vi "set_smith_axis_label.vi"(4 "r/x_scale":bool, 5 "left_center":dbl=300.0, 6 "show_z":bool=TRUE, 7 "top_center":dbl=300.0, 8 "Z50":dbl=50.0, 9 "x":dbl[](array[numeric])=[0.2, 0.4, 0.6, 0.8, 1.0, 1.2, 1.6, 2.0, 3.0, 5.0, -0.2, -0.4, -0.6, -0.8, -1.0, -1.2, -1.6, -2.0, -3.0, -5.0], 10 "r":dbl[](array[numeric])=[0.0, 0.1, 0.2, 0.3, 0.5, 0.7, 1.0, 1.4, 2.0, 3.0, 5.0, 10.0, 20.0], 11 "smith_in":picture) -> (3 "smith_out":picture)   [LabVIEW 2025]
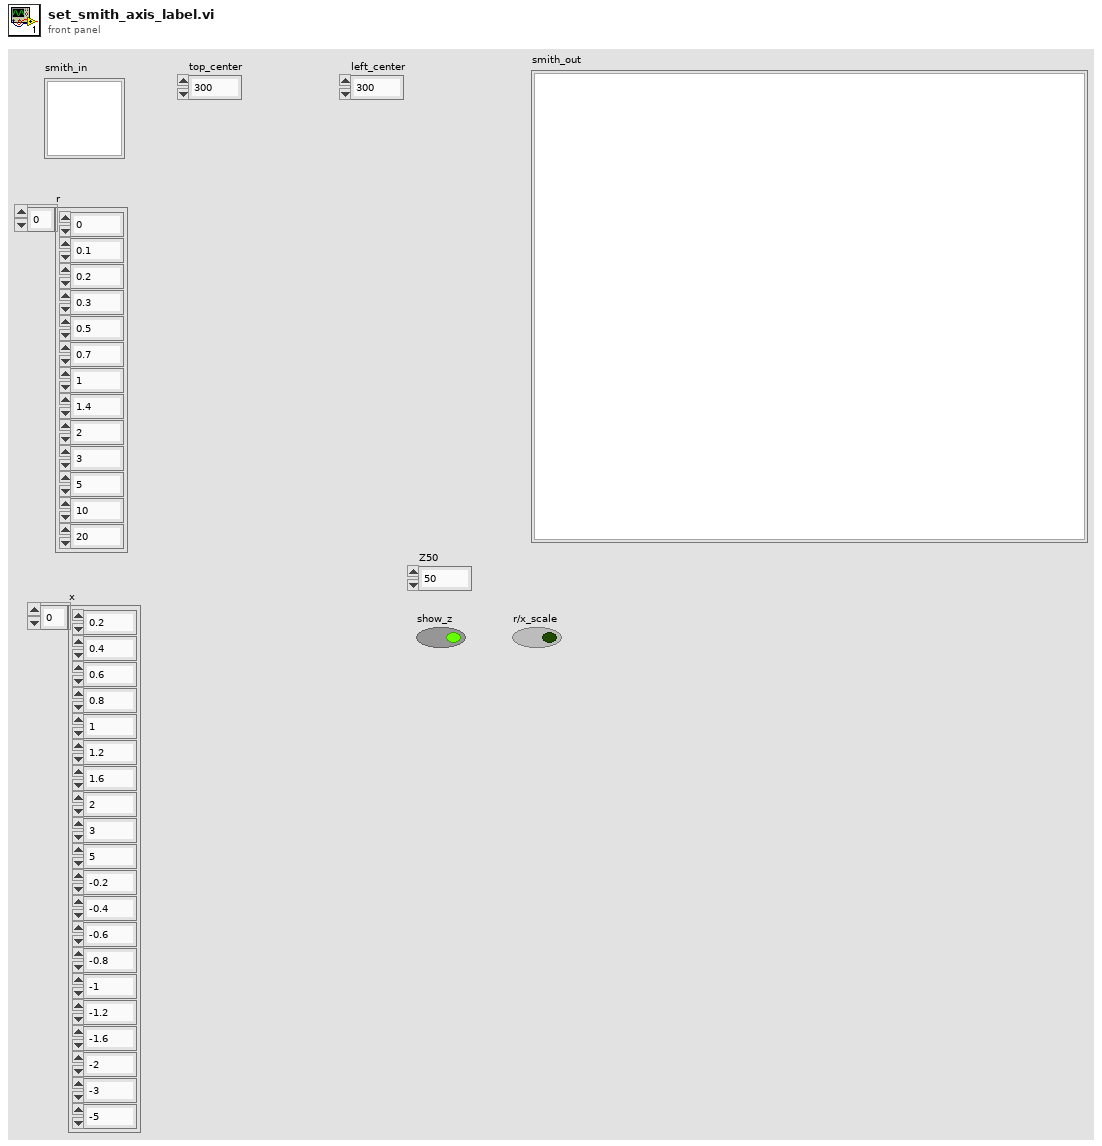
[diagram p1: front panel]
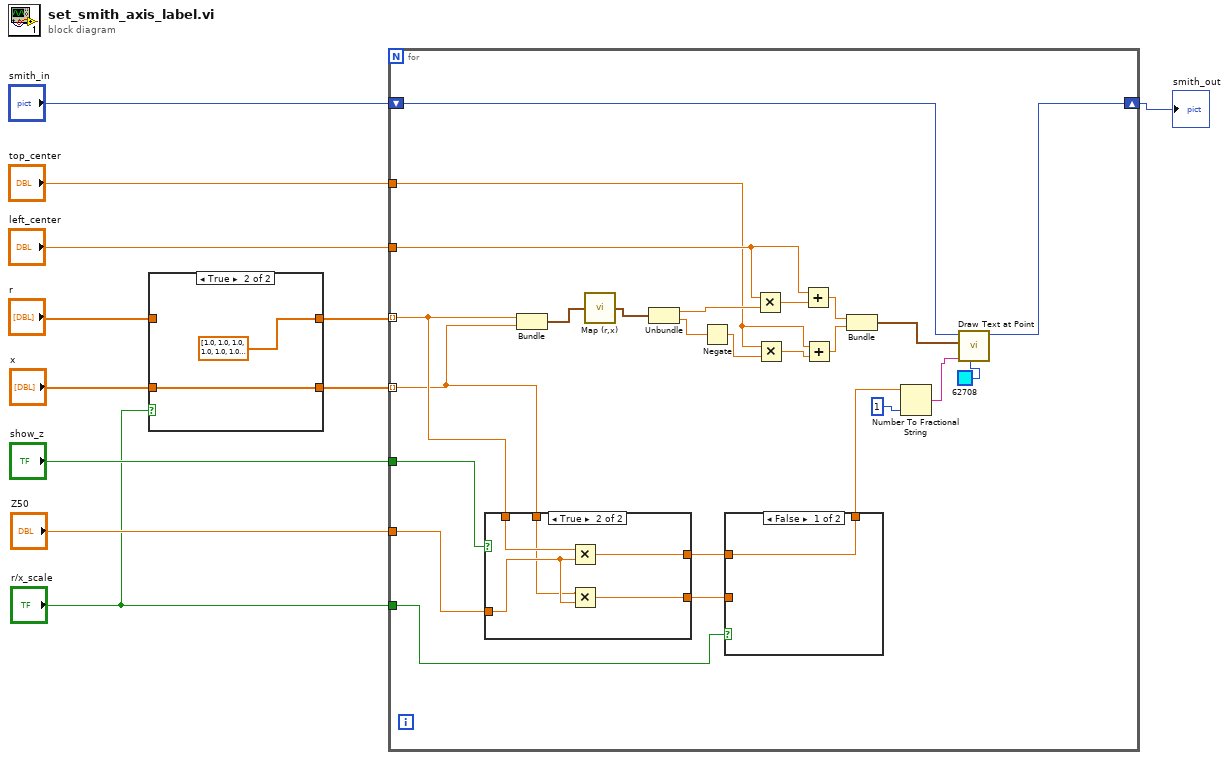
[diagram p0: block diagram]
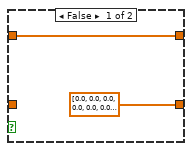
[diagram p2: hidden frame]
diagram:
  n1 = case shown="True" "r/x_scale" {
    tunnel: [w13 dbl[] [1.0, 1.0, 1.0, 1.0, 1.0, 1.0, 1.0, 1.0, 1.0, 1.0, 1.0, 1.0, 1.0, 1.0, 1.0, 1.0, 1.0, 1.0, 1.0, 1.0] ("r")] -> w4
    tunnel: "r" -> [w13 _]
    tunnel: [dbl[] [0.0, 0.0, 0.0, 0.0, 0.0, 0.0, 0.0, 0.0, 0.0, 0.0, 0.0, 0.0, 0.0] ("r") w15] -> w2
    tunnel: "x" -> [_ w15]
    frame False {
    }
    frame True {
    }
  }
  n2 = for {
    tunnel: w4 -> [w17] mode=indexing
    tunnel: "left_center" -> [w31]
    tunnel: "top_center" -> [w30]
    shift-right: [w26] -> w9
    shift-left: "smith_in" -> [w27]
    tunnel: w2 -> [w16] mode=indexing
    tunnel: "show_z" -> [w23]
    tunnel: "Z50" -> [w22]
    tunnel: "r/x_scale" -> [w18]
    n3 = case shown="True" w23 {
      tunnel: w22 -> [_ w47]
      tunnel: w17 -> [w44 w49]
      tunnel: [w44 w48] -> w20
      tunnel: w16 -> [w43 w46]
      tunnel: [w43 w45] -> w19
      frame False {
      }
      frame True {
        n4 = Multiply(x=w49, y=w47) -> (x*y=w48:dbl)
        n5 = Multiply(x=w46, y=w47) -> (x*y=w45:dbl)
      }
    }
    n6 = Bundle(w17, w16) -> (w40:cluster{dbl, dbl})  [unwired: 1 in]
    n7 = call <vilib>:"Map (r,x).VI"("Smith Pt"=w40) -> ("Point (h,v)"=w33:cluster{"horizontal":dbl, "vertical":dbl})
    n8 = Unbundle(w33) -> ("horizontal"=w32:dbl, "vertical"=w39:dbl)
    n9 = Negate(x=w39) -> (-x=w38:dbl)
    n10 = case shown="False" w18 {
      tunnel: [w41 w42] -> w21
      tunnel: w20 -> [w41 _]
      tunnel: w19 -> [_ w42]
      frame False {
      }
      frame True {
      }
    }
    n11 = Multiply(x=w31, y=w32) -> (x*y=w34:dbl)
    n12 = Multiply(x=w30, y=w38) -> (x*y=w36:dbl)
    n13 = Add(x=w31, y=w34) -> (x+y=w35:dbl)
    n14 = Add(x=w30, y=w36) -> (x+y=w37:dbl)
    n15 = Bundle(w35, w37) -> (w28:cluster{dbl, dbl})  [unwired: 1 in]
    n16 = Number To Fractional String(number=w21, precision (6)=i16 1) -> (F-format string=w24:string)  [unwired: 2 in]
    n17 = call <vilib>:"Draw Text at Point.vi"("text color(black)"=u32 62708, "text"=w24, "origin"=w28, "picture"=w27) -> ("new picture"=w26:picture)  [unwired: 6 in, 1 out]
  }
  "smith_out" <- w9
